vi "sendOutputData.vi"(8 "error in (no error)":errorcluster, 11 "Model in":refnum<class "Model.lvclass">) -> (0 "error out":errorcluster, 3 "Model out":refnum<class "Model.lvclass">)   [LabVIEW 2015, in "Model.lvclass"]
uses:
  Model.lvclass
  Model.lvclass/Model.ctl
  <userlib>/Common/ILC/ILC/ILC.lvclass/ILC.ctl
  <userlib>/Common/ILC/ILC/ILC.lvclass
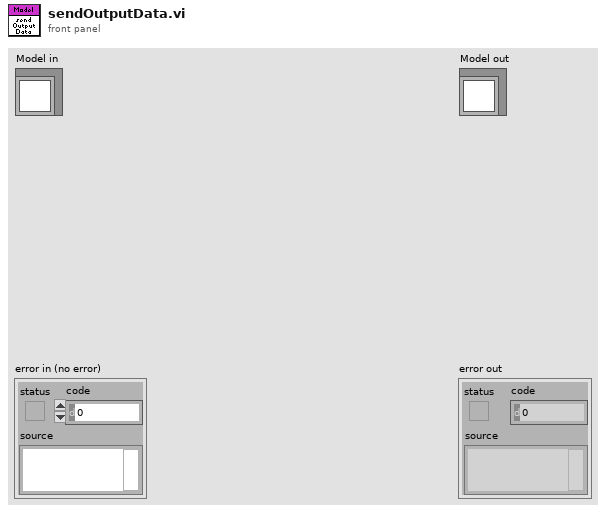
[diagram p1: front panel]
types:
  T1 = typedef "ILCCommon.lvlib/ILCTypedefs.lvlib/OutputData.ctl" = cluster{"Step & Direction":i16, "Blower RPM":u8, "PWM (SSR)":u8, "Ch1":u16, "Ch2":u16, "Ch3":u16, "Ch4":u16}
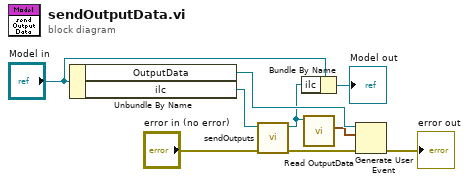
[diagram p0: block diagram]
diagram:
  n1 = Unbundle By Name("Model in") -> ("OutputData"=w9:refnum<user-event>, "ilc"=w5:refnum<class "ILC.lvclass">)
  n2 = call <userlib>:"sendOutputs.vi"("error in (no error)"="error in (no error)", "ILC in"=w5) -> ("error out"=w3:errorcluster, "ILC out"=w2:refnum<class "ILC.lvclass">)  [unwired: 8 in]
  n3 = Bundle By Name(cluster="Model in", "ilc"=w2) -> (→"Model out":refnum<class "Model.lvclass">)
  n4 = call <userlib>:"Read OutputData.vi"("ILC in"=w2) -> ("OutputData"=w1:T1)  [unwired: 9 in, 1 out]
  n5 = Generate User Event(user event=w9, event data cluster=w1, error in=w3) -> (error out=→"error out":errorcluster)  [unwired: 1 in, 1 out]
